vi "Pulse Parameter Calculation.vi"(8 "error in":errorcluster, 11 "NewVal":T1={"Preliminary Settings"={"Nº of Scans (ns)"=3, "Pulse Frequency"=10000000.0}, "Detlay Settings"={"Delay d1"=10.0, "Delay d2"=0.0, "d1 Units"=enum."ms", "d2 Units 2"=enum."ms"}, "Pulse Settings"={"Duration Signal P1"=20.0, "Power Level P1"=1023, "Phase"=90, "Duration Units"=enum."ms"}, "Acquisition Settings"={"Number Samples"=2000, "Time Between Points"=0.0, "Time Units"=enum."ms"}} {"Acquisition Settings"."Time Between Points" min=0.0 step=1.0; "Acquisition Settings"."Number Samples" step=1; "Pulse Settings"."Phase" max=270 step=90; "Pulse Settings"."Power Level P1" max=1023 step=1; "Pulse Settings"."Duration Signal P1" min=0.0 step=1.0; "Detlay Settings"."Delay d2" min=0.0 step=1.0; "Detlay Settings"."Delay d1" min=0.0 step=1.0; "Preliminary Settings"."Pulse Frequency" min=1.0 format="%^#_6e"; "Preliminary Settings"."Nº of Scans (ns)" step=1}) -> (0 "error out":errorcluster, 3 "x*y":dbl)   [LabVIEW 2011]
uses:
  Controls/90 Degree Pulse Settings.ctl
  Controls/Preliminary Settings.ctl
  Controls/Delay Settings.ctl
  Controls/Pulse Settings.ctl
  Controls/Acquisition Settings.ctl
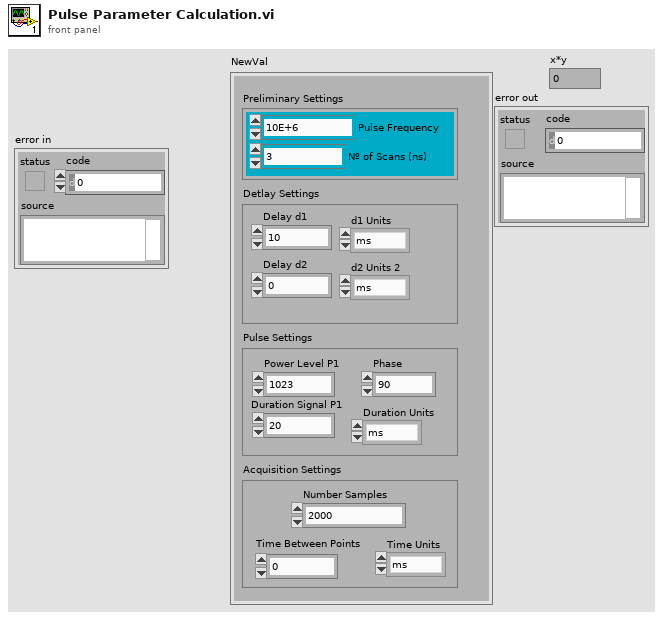
[diagram p1: front panel]
types:
  T1 = typedef "90 Degree Pulse Settings.ctl" = cluster{"Preliminary Settings":T2, "Detlay Settings":T3, "Pulse Settings":T4, "Acquisition Settings":T5}
  T2 = typedef "Preliminary Settings.ctl" = cluster{"Nº of Scans (ns)":u16, "Pulse Frequency":dbl}
  T3 = typedef "Delay Settings.ctl" = cluster{"Delay d1":dbl, "Delay d2":dbl, "d1 Units":enum16{"ms", "us"}, "d2 Units 2":enum16{"ms", "us"}}
  T4 = typedef "Pulse Settings.ctl" = cluster{"Duration Signal P1":dbl, "Power Level P1":u16, "Phase":u16, "Duration Units":enum16{"ms", "us"}}
  T5 = typedef "Acquisition Settings.ctl" = cluster{"Number Samples":u16, "Time Between Points":dbl, "Time Units":enum16{"ms", "us"}}
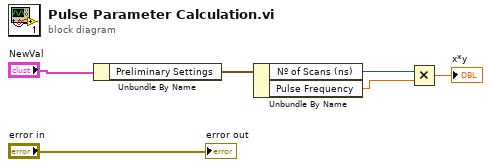
[diagram p0: block diagram]
diagram:
  n1 = Unbundle By Name("NewVal") -> ("Preliminary Settings"=w5:T2)
  n2 = Unbundle By Name(w5) -> ("Nº of Scans (ns)"=w4:u16, "Pulse Frequency"=w3:dbl)
  n3 = Multiply(x=w4, y=w3) -> (x*y=→"x*y":dbl)
  "error out" <- "error in"
